vi "JSON Tree View.vi"(8 "error in (no error)":errorcluster, 10 "JSON Tree Expanded Reference":refnum<vi>, 11 "JSON Tree":variant) -> (0 "error out":errorcluster, 3 "JSON Tree Passthrough":variant)   [LabVIEW 2013, in "i3-json.lvlib"]
doc: "Use this template to build a VI to use as a subVI."
uses:
  i3-json.lvlib
  JSON Tree View Files/Tree Nodes.ctl
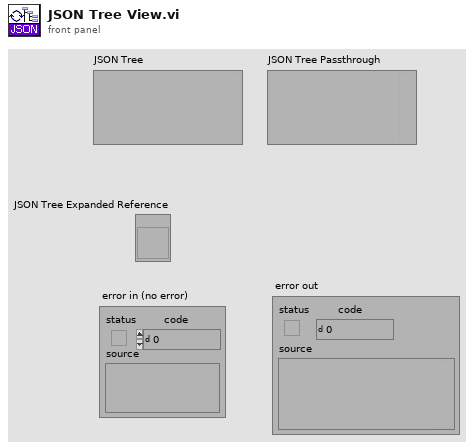
[diagram p1: front panel]
types:
  T1 = typedef "i3-json.lvlib/Tree Nodes.ctl" = cluster{"Left Cell String":string, "Child Text":string[], "Child Tag":string, "Item Indent":i32, "Child Only?":bool, "Glyph Index":i32}
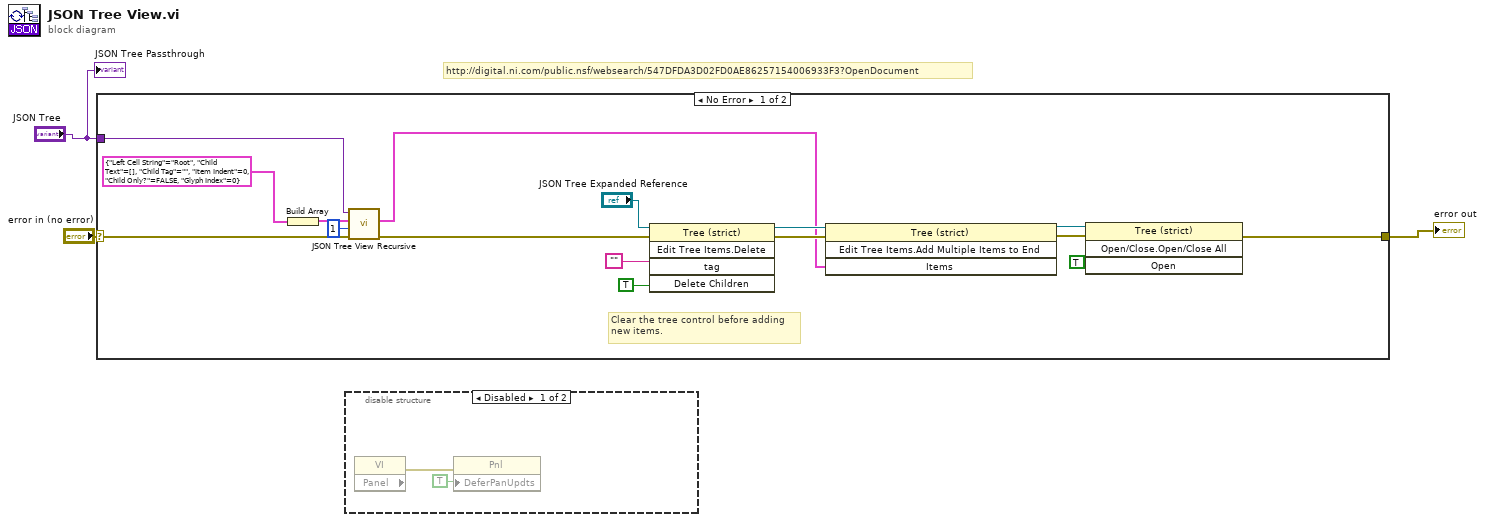
[diagram p0: block diagram]
diagram:
  # "http://digital.ni.com/public.nsf/websearch/547DFDA3D02FD0AE86257154006933F3?OpenDocument"
  n1 = case shown="No Error" "error in (no error)" {
    selector: "error in (no error)" -> [w19 w20]
    tunnel: [w5 w20] -> w2
    tunnel: "JSON Tree" -> [w4 _]
    frame No Error {
      # "Clear the tree control before adding\nnew items."
      n2 = Build Array(T1 {"Left Cell String"="Root", "Child Text"=[], "Child Tag"="", "Item Indent"=0, "Child Only?"=FALSE, "Glyph Index"=0} ("Item")) -> (w17:T1[])
      n3 = call "JSON Tree View Recursive.vi"("error in (no error)"=w19, "Item Indent In"=1, "JSON Tree Expanded In"=w17, "JSON Tree"=w4) -> ("error out"=w6:errorcluster, "JSON Tree Expanded Out"=w11:T1[])  [unwired: 5 in]
      n4 = invoke class="Tree (strict)" method="Edit Tree Items.Delete"(reference="JSON Tree Expanded Reference", error in=w6, "tag"="", "Delete Children"=TRUE ("Delete Children?")) -> (reference out=w12:refnum<vi>, error out=w13:errorcluster)  [unwired: 1 in, 3 out]
      n5 = invoke class="Tree (strict)" method="Edit Tree Items.Add Multiple Items to End"(reference=w12, error in=w13, "Items"=w11) -> (reference out=w9:refnum<vi>, error out=w10:errorcluster)  [unwired: 1 in, 2 out]
      n6 = invoke class="Tree (strict)" method="Open/Close.Open/Close All"(reference=w9, error in=w10, "Open"=TRUE ("Open?")) -> (error out=w5:errorcluster)  [unwired: 1 in, 3 out]
    }
    frame Error {
    }
  }
  "error out" <- w2
  n7 = disable-structure shown="Disabled" {
    frame Disabled {
      n8 = property class="VI"() -> (error out=w21:errorcluster, "Panel"=w23:refnum<vi>)  [unwired: 2 in, 1 out]
      n9 = property class="Pnl"(error in=w21, "DeferPanUpdts"=TRUE ("Defer Panel Updates")) -> ()  [unwired: 1 in, 2 out]
    }
    frame Enabled {
    }
  }
  "JSON Tree Passthrough" <- "JSON Tree"
